vi "PutInstrument.vi"(8 "error in (no error)":errorcluster, 10 "InstrumentPut":T1, 11 "ByteGSWebAPI-V0 in":refnum<class "ByteGSWebAPI-V0.lvclass">) -> (0 "error out":errorcluster, 3 "ByteGSWebAPI-V0 out":refnum<class "ByteGSWebAPI-V0.lvclass">, 4 "body":string, 6 "headers":string)   [LabVIEW 2019, in "ByteGSWebAPI-V0.lvclass"]
uses:
  ByteGSWebAPI-V0.lvclass
  Cntrls/SingleInstrument.ctl
  c2a64cc6-83f8-4dd7-87c5-b1adee6936e4.vi
  <vilib>/JDP Science/JSONtext/Variant to JSON Text.vi
  <vilib>/JDP Science/JSONtext/LVClass Serializer/JSONtext LVClass Serializer.lvclass
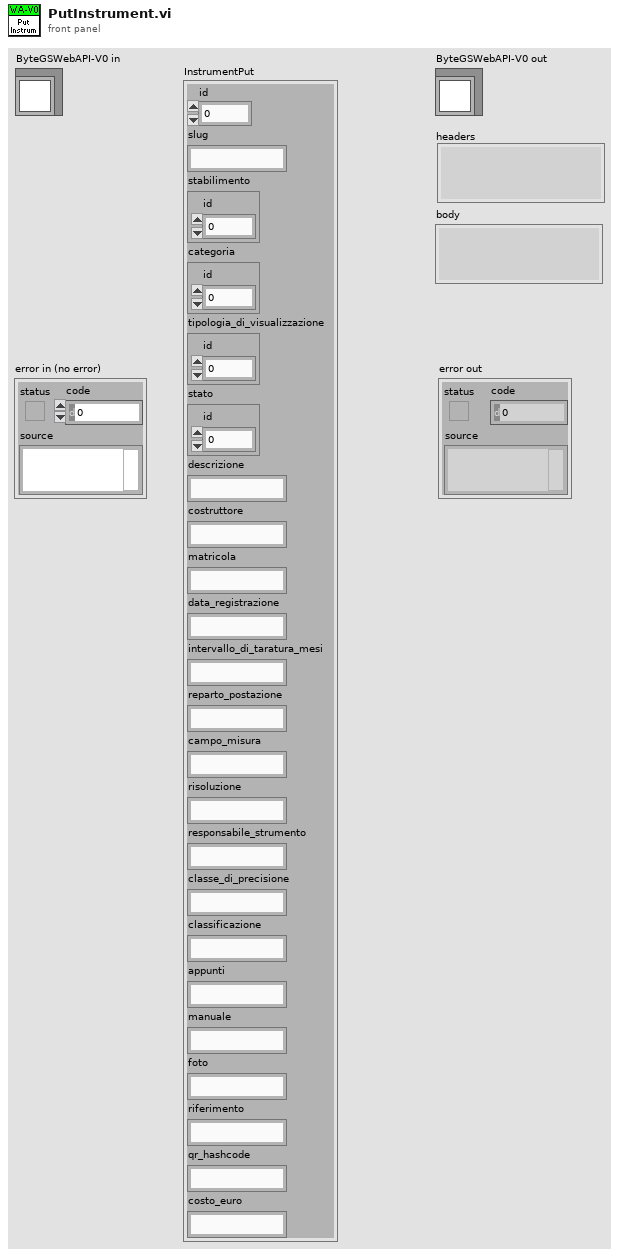
[diagram p1: front panel]
types:
  T1 = typedef "ByteGSWebAPI-V0.lvclass/SingleInstrument.ctl" = cluster{"id":i32, "slug":string, "stabilimento":cluster{"id":dbl}, "categoria":cluster{"id":dbl}, "tipologia_di_visualizzazione":cluster{"id":dbl}, "stato":cluster{"id":dbl}, "descrizione":string, "costruttore":string, "matricola":string, "data_registrazione":string, "intervallo_di_taratura_mesi":string, "reparto_postazione":string, "campo_misura":string, "risoluzione":string, "responsabile_strumento":string, "classe_di_precisione":string, "classificazione":string, "appunti":string, "manuale":string, "foto":string, "riferimento":string, "qr_hashcode":string, "costo_euro":string}
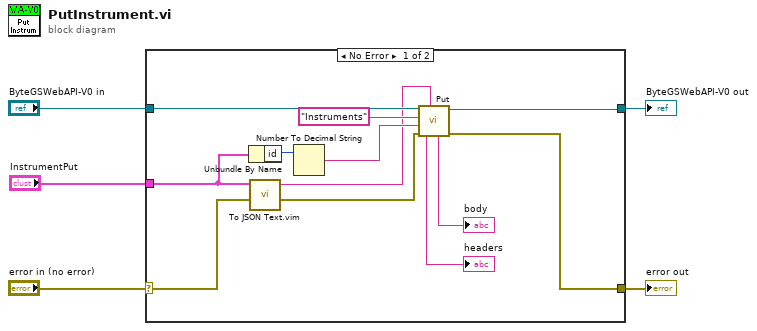
[diagram p0: block diagram]
diagram:
  n1 = case shown="No Error" "error in (no error)" {
    selector: "error in (no error)" -> [w17 w19]
    tunnel: [w6 w19] -> w4
    tunnel: [w13 w18] -> w2
    tunnel: "ByteGSWebAPI-V0 in" -> [w14 w18]
    tunnel: "InstrumentPut" -> [w15 _]
    frame No Error {
      n2 = Unbundle By Name(w15) -> ("id"=w12:i32)
      n3 = call "To JSON Text.vim"("error in (no error)"=w17, "Anything"=w15) -> ("error out"=w7:errorcluster, "<JSON>"=w8:string)  [unwired: 8 in]
      n4 = Number To Decimal String(number=w12) -> (decimal integer string=w11:string)  [unwired: 1 in]
      n5 = call "Put.vi"("PutRequest"=w8, "error in (no error)"=w7, "Parameter"=w11, "Request"="Instruments", "ByteGSWebAPI-V0 in"=w14) -> ("error out"=w6:errorcluster, "ByteGSWebAPI-V0 out"=w13:refnum<class "ByteGSWebAPI-V0.lvclass">, "body"=→"body":string, "headers"=→"headers":string)  [unwired: 3 in]
    }
    frame Error {
    }
  }
  "error out" <- w4
  "ByteGSWebAPI-V0 out" <- w2
